vi "SwissSPAD Live_Get-Set Saving Tasks Information.vi"(6 "Get (F)/Set":bool, 8 "error in (no error)":errorcluster, 9 "# New Images Saved (1)":i32=1, 10 "# Images (Total)":i32=-1, 11 "File Path::n":string) -> (0 "error out":errorcluster, 1 "Complete Saving Task Information":T1, 2 "# Saving Tasks":i32=-1, 3 "Array of Saving Tasks Information":T1[](array[typedef]))   [LabVIEW 2021]
doc: "File Path: provided when created only\n# Images (Total): also provided when a new file is added, otherwise ignored\nNew Image Saved (1): how many images are added to the file (default: 1)"
uses:
  SwissSPAD Live_File Saving Task Information.ctl
  SwissSPAD Live_Internal Data List.ctl
  Variant/Variant to Data/Variant to Data.lvlib
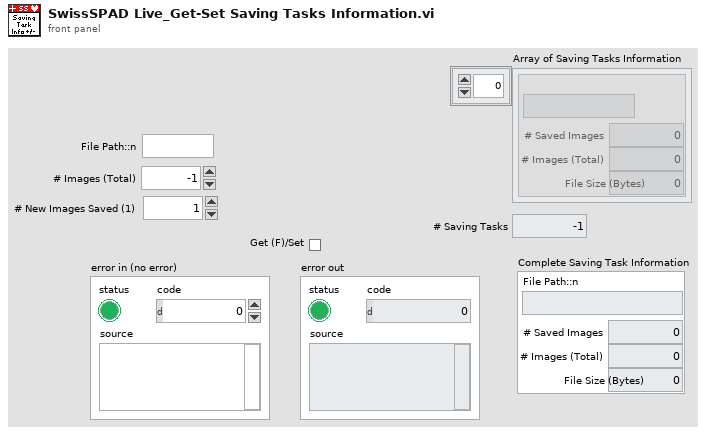
[diagram p1: front panel]
types:
  T1 = typedef "SwissSPAD Live_File Saving Task Information.ctl" = cluster{"File Path::n":string, "# Saved Images":i32, "# Images (Total)":i32, "File Size (Bytes)":i64}
  T2 = typedef "SwissSPAD Live_Internal Data List.ctl" = enum16{"Number of pending file saving tasks", "File Saving Tasks Information", "Current Image ROI Information", "# FPGA Reset Attempts", "Histogram Cursor Locations", "Histogram Window is Open"}
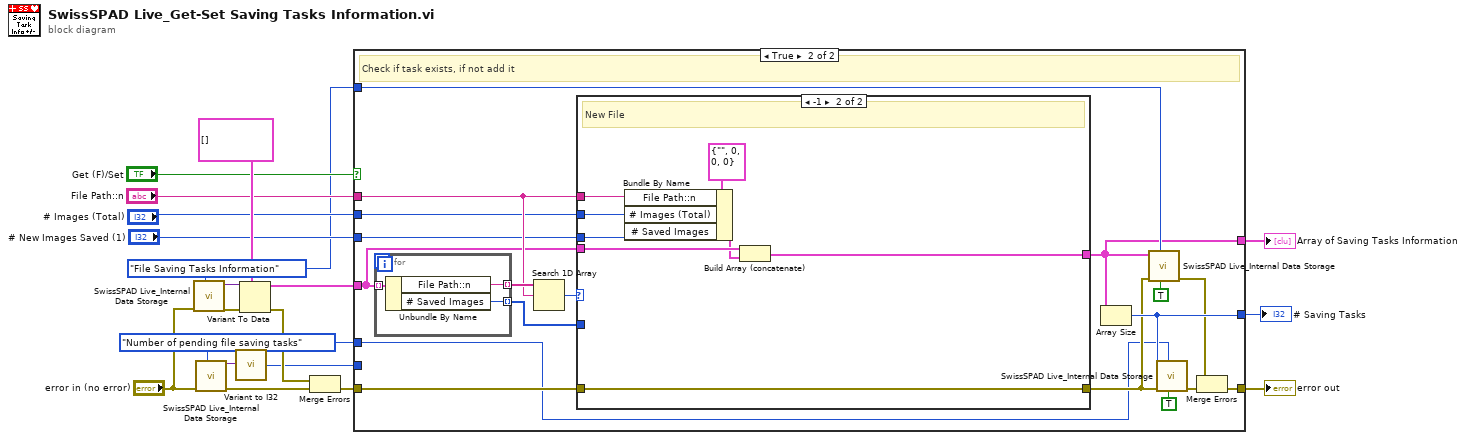
[diagram p0: block diagram]
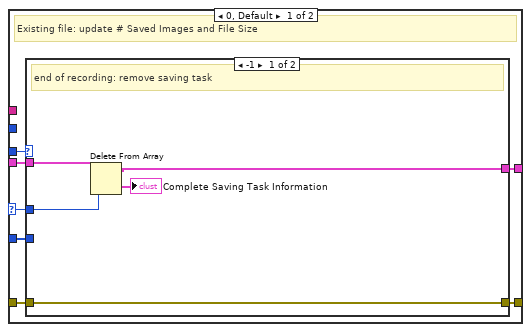
[diagram p3: hidden frame]
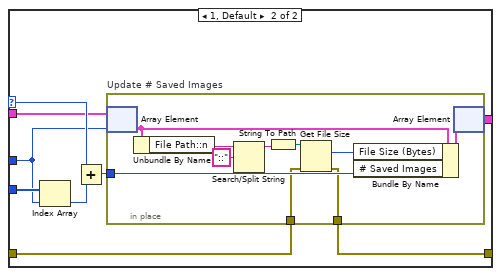
[diagram p4: hidden frame]
diagram:
  w1 = SwissSPAD_Live_Internal_Data_List."File Saving Tasks Information" ("SS2 Live Data")
  w2 = SwissSPAD_Live_Internal_Data_List."Number of pending file saving tasks" ("SS2 Live Data")
  n1 = call "SwissSPAD Live_Internal Data Storage.vi"("SS2 Live Data"=w1, "Error In"="error in (no error)") -> ("Error Out"=w15:errorcluster, "Variant"=w16:variant)  [unwired: 7 in, 1 out]
  n2 = call "SwissSPAD Live_Internal Data Storage.vi"("SS2 Live Data"=w2, "Error In"="error in (no error)") -> ("Error Out"=w17:errorcluster, "Variant"=w13:variant)  [unwired: 7 in, 1 out]
  n3 = call "Variant to I32.vi"("Variant"=w13) -> ("Value"=w9:i32)  [unwired: 8 in]
  n4 = Variant To Data(error in=w15, type=T1[] [] ("Array of Saving Tasks Information"), Variant=w16) -> (data=w12:T1[], error out=w14:errorcluster)
  n5 = Merge Errors(w14, w17) -> (w4:errorcluster)
  n6 = case shown="True" "Get (F)/Set" {
    tunnel: w12 -> [w22 w34]
    tunnel: [w22 w27] -> w10
    tunnel: w9 -> [w21 _]
    tunnel: [w21 w32] -> w5
    tunnel: "File Path::n" -> [_ w37]
    tunnel: "# Images (Total)" -> [_ w36]
    tunnel: "# New Images Saved (1)" -> [_ w35]
    tunnel: w4 -> [w20 w33]
    tunnel: [w20 w25] -> w3
    tunnel: w2 -> [_ w23]
    tunnel: w1 -> [_ w28]
    frame False {
    }
    frame True {
      # "Check if task exists, if not add it"
      n7 = for {
        tunnel: w34 -> [w82] mode=indexing
        tunnel: [w81] -> w40 mode=indexing
        tunnel: [w80] -> w39 mode=indexing
        n8 = Unbundle By Name(w82) -> ("File Path::n"=w81:string, "# Saved Images"=w80:i32)
      }
      n9 = Search 1D Array(1D array=w40, element=w37) -> (index of element=w38:i32)  [unwired: 1 in]
      n10 = case shown="-1" w38 {
        selector: w38 -> [w43 _]
        tunnel: w39 -> [w47 _]
        tunnel: w37 -> [_ w78]
        tunnel: w36 -> [_ w77]
        tunnel: w35 -> [w46 w73]
        tunnel: w34 -> [w45 w76]
        tunnel: [w44 w74] -> w27
        tunnel: w33 -> [w42 w72]
        tunnel: [w41 w72] -> w29
        frame 0, Default {
          # "Existing file: update # Saved Images and File Size"
          n11 = case shown="-1" w46 {
            selector: w46 -> [_ w60]
            tunnel: w47 -> [_ w61]
            tunnel: w45 -> [w52 w58]
            tunnel: [w50 w56] -> w44
            tunnel: w43 -> [w51 w55]
            tunnel: w42 -> [w48 w54]
            tunnel: [w48 w53] -> w41
            frame -1 {
              # "end of recording: remove saving task"
              n12 = Delete From Array(array=w52, index=w51) -> (deleted portion=→"Complete Saving Task Information":T1, array with subset deleted=w50:T1[])  [unwired: 1 in]
            }
            frame 1, Default {
              n13 = Index Array(array=w61, index=w55) -> (element=w59:i32)
              n14 = Add(x=w60, y=w59) -> (x+y=w57:i32)
              n15 = in-place "Update # Saved Images" {
                in-place-border: w57 -> [w69]
                in-place-border: w54 -> [w67]
                in-place-border: [w65] -> w53
                n16 = in-place-array #1(w58, w55) -> (w71:T1)
                n17 = Unbundle By Name(w71) -> ("File Path::n"=w64:string)
                n18 = Search/Split String(string=w64, search string/char (-)="::") -> (substring before match=w63:string)  [unwired: 1 in, 2 out]
                n19 = String To Path(string=w63) -> (path=w68:path)
                n20 = Get File Size(file=w68, error in=w67) -> (size (in bytes)=w66:i64, 0:w65:errorcluster)  [unwired: 1 out]
                n21 = Bundle By Name(cluster=w71, "File Size (Bytes)"=w66, "# Saved Images"=w69) -> (w70:T1)
                n22 = in-place-array #1(w70) -> (w56:T1[])  [unwired: 1 out]
              }
            }
          }
        }
        frame -1 {
          # "New File"
          n23 = Bundle By Name(cluster=T1 {"File Path::n"="", "# Saved Images"=0, "# Images (Total)"=0, "File Size (Bytes)"=0} ("File Saving Task Information"), "File Path::n"=w78, "# Images (Total)"=w77, "# Saved Images"=w73) -> (w75:T1)
          n24 = Build Array (concatenate)(w76, w75) -> (w74:T1[])
        }
      }
      n25 = Array Size(array=w27) -> (size(s)=w32:i32)
      n26 = call "SwissSPAD Live_Internal Data Storage.vi"("Get(F)/Set"=TRUE, "SS2 Live Data"=w28, "Error In"=w29, "Variant"=w27) -> ("Error Out"=w24:errorcluster)  [unwired: 5 in, 2 out]
      n27 = call "SwissSPAD Live_Internal Data Storage.vi"("Get(F)/Set"=TRUE, "SS2 Live Data"=w23, "Error In"=w29, "Variant"=w32) -> ("Error Out"=w31:errorcluster)  [unwired: 5 in, 2 out]
      n28 = Merge Errors(w24, w31) -> (w25:errorcluster)
    }
  }
  "error out" <- w3
  "# Saving Tasks" <- w5
  "Array of Saving Tasks Information" <- w10
